vi "MapSelect.vi"(10 "Scan Control":string(combo)="Honeycomb" caption="Combo Box") -> (2 "Map":string)   [LabVIEW 2023]
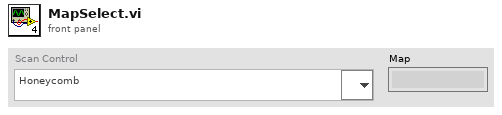
[diagram p1: front panel]
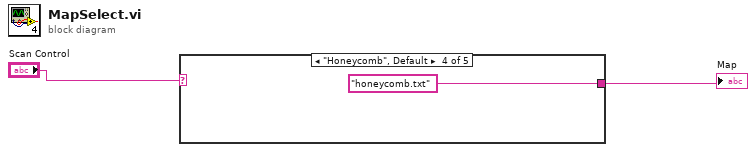
[diagram p0: block diagram]
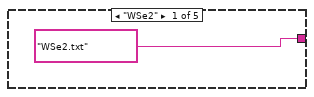
[diagram p2: hidden frame]
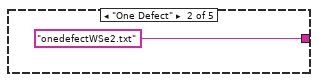
[diagram p3: hidden frame]
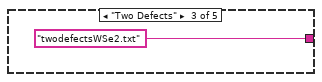
[diagram p4: hidden frame]
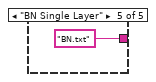
[diagram p5: hidden frame]
diagram:
  n1 = case shown="\"Honeycomb\", Default" "Scan Control" {
    tunnel: ["WSe2.txt" "onedefectWSe2.txt" "twodefectsWSe2.txt" "honeycomb.txt" "BN.txt"] -> w1
    frame "WSe2" {
    }
    frame "One Defect" {
    }
    frame "Two Defects" {
    }
    frame "Honeycomb", Default {
    }
    frame "BN Single Layer" {
    }
  }
  "Map" <- w1
